vi "Shift_003.vi"() -> ()   [LabVIEW 2019]
panel:
  out "a":cluster{dbl[unit][], dbl[unit][]}(graph)
  out "v":cluster{dbl[unit][], dbl[unit][]}(graph)
  out "x":cluster{dbl[unit][], dbl[unit][]}(graph)
  out "time (tk)":dbl[unit][](array[numeric])
  out "a":dbl[unit][](graph)
  out "v":dbl[unit][](graph)
  out "x":dbl[unit][](graph)
  out "x(tk)":dbl[unit][](array[numeric])
  out "v(tk)":dbl[unit][](array[numeric])
  out "a(k)":dbl[unit][](array[numeric])
  in  "M":dbl[unit]=100.0
  in  "k":dbl[unit]=1000.0
  in  "v0":dbl[unit]
  in  "x0":dbl[unit]=2.0
  in  "Dt":dbl[unit]=1e-05
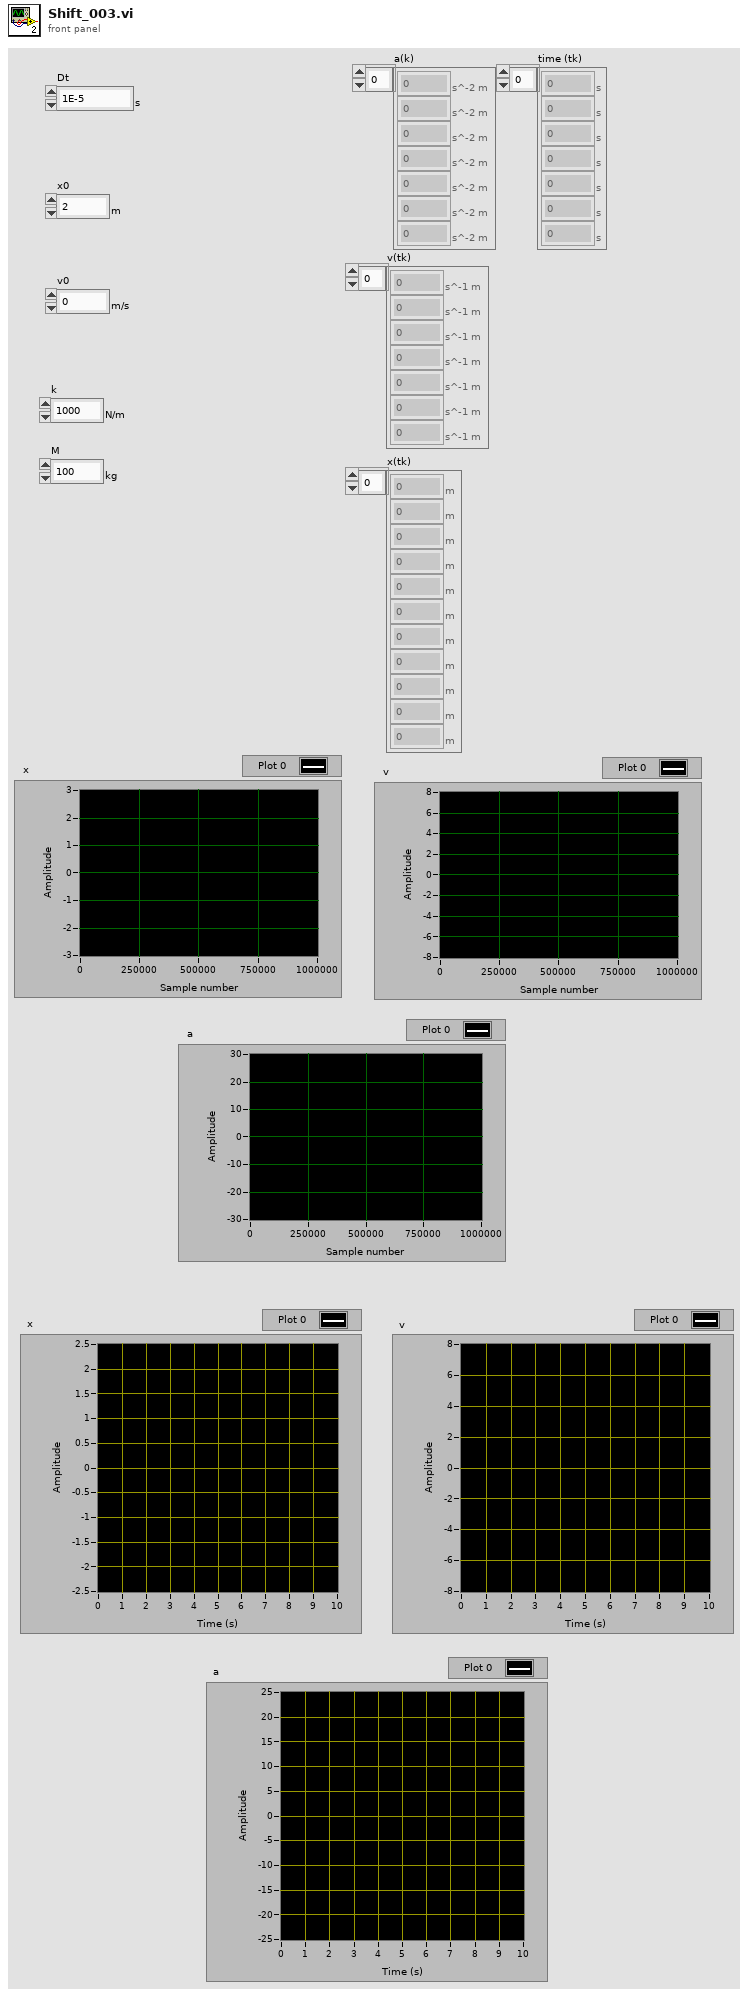
[diagram p1: front panel]
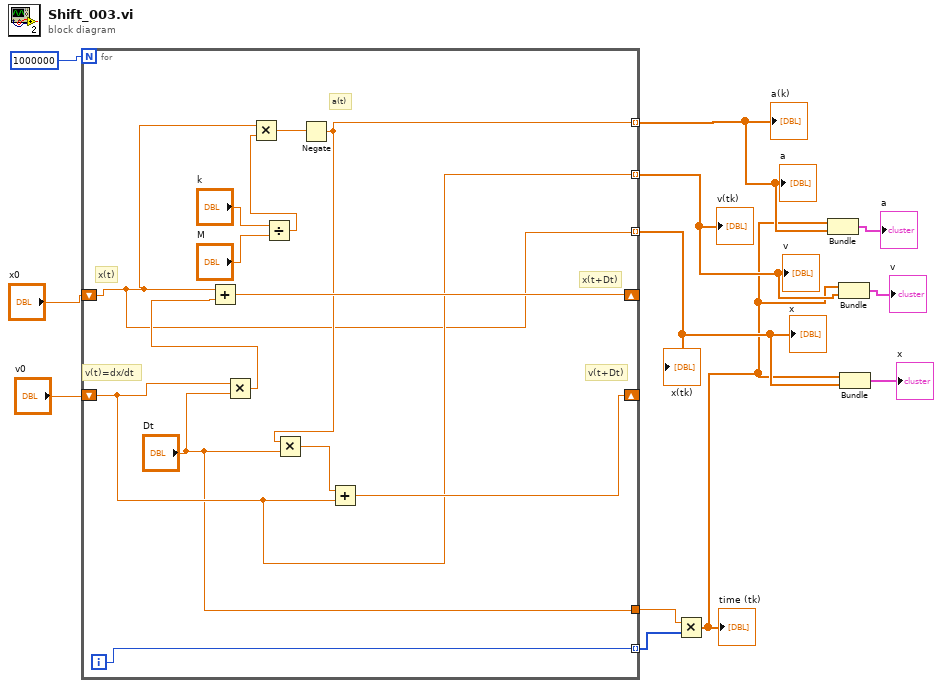
[diagram p0: block diagram]
diagram:
  n1 = for {
    N: 1000000 -> [_]
    shift-right: [w24] -> _
    shift-left: "x0" -> [w15]
    shift-right: [w18] -> _
    shift-left: "v0" -> [w16]
    tunnel: [w17] -> w4 mode=indexing
    tunnel: [w16] -> w3 mode=indexing
    tunnel: [w15] -> w2 mode=indexing
    tunnel: [w14] -> w8 mode=indexing
    tunnel: ["Dt"] -> w9
    i -> [w14]
    # "a(t)"
    # "v(t+Dt)"
    # "x(t+Dt)"
    # "v(t)=dx/dt"
    # "x(t)"
    n2 = Multiply(x=w16, y="Dt") -> (x*y=w25:dbl[unit])
    n3 = Add(x=w15, y=w25) -> (x+y=w24:dbl[unit])
    n4 = Divide(x="k", y="M") -> (x/y=w21:dbl[unit])
    n5 = Multiply(x=w15, y=w21) -> (x*y=w20:dbl[unit])
    n6 = Negate(x=w20) -> (-x=w17:dbl[unit])
    n7 = Multiply(x=w17, y="Dt") -> (x*y=w19:dbl[unit])
    n8 = Add(x=w19, y=w16) -> (x+y=w18:dbl[unit])
  }
  "a(k)" <- w4
  "v(tk)" <- w3
  "x(tk)" <- w2
  "v" <- w3
  "a" <- w4
  "x" <- w2
  n9 = Multiply(x=w9, y=w8) -> (x*y=w1:dbl[unit][])
  "time (tk)" <- w1
  n10 = Bundle(w1, w4) -> (→"a":cluster{dbl[unit][], dbl[unit][]})  [unwired: 1 in]
  n11 = Bundle(w1, w3) -> (→"v":cluster{dbl[unit][], dbl[unit][]})  [unwired: 1 in]
  n12 = Bundle(w1, w2) -> (→"x":cluster{dbl[unit][], dbl[unit][]})  [unwired: 1 in]
